vi "Filter.vi"(8 "error in (no error)":errorcluster, 10 "Selected Runnables":string[](array[string]), 11 "LUnit Test Case V2 In":refnum<class "LUnit Test Case V2.lvclass">) -> (0 "error out":errorcluster, 3 "LUnit Test Case V2 Out":refnum<class "LUnit Test Case V2.lvclass">)   [LabVIEW 2020, in "LUnit Test Case V2.lvclass"]
uses:
  LUnit Test Case V2.lvclass
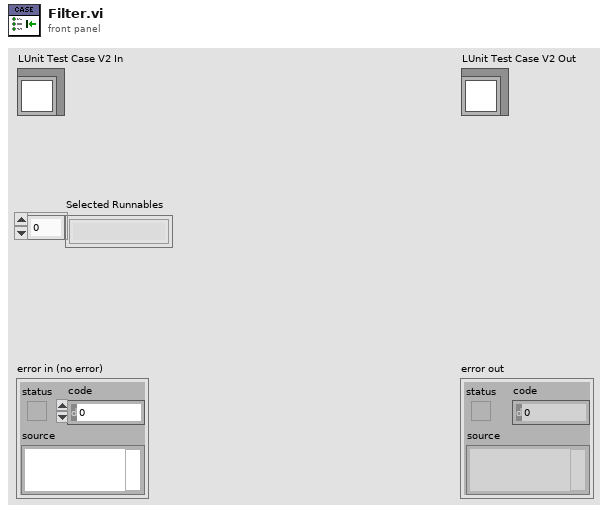
[diagram p1: front panel]
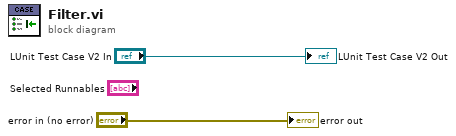
[diagram p0: block diagram]
diagram:
  "error out" <- "error in (no error)"
  "LUnit Test Case V2 Out" <- "LUnit Test Case V2 In"
